vi "load_class-file.vi"(8 "error in (no error)":errorcluster, 11 "class_path":path) -> (0 "error out":errorcluster)   [LabVIEW 2015, in "lv-dialog.lvlib" / "v1.lvlib"]
uses:
  v1.lvlib
  private/_controls/fg_command.ctl
  class/v1.lvclass
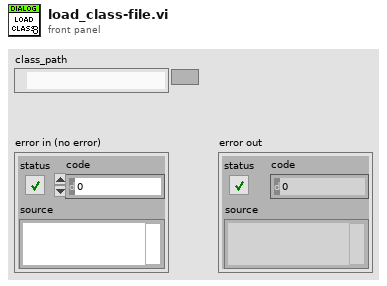
[diagram p1: front panel]
types:
  T1 = typedef "lv-dialog.lvlib/v1.lvlib/fg_command.ctl" = enum16{"null", "initialize", "read", "write", "shutdown"}
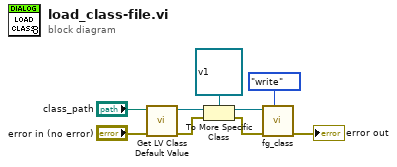
[diagram p0: block diagram]
diagram:
  n1 = call <vilib>:"Get LV Class Default Value.vi"("error in (no error)"="error in (no error)", "class path"="class_path") -> ("error out"=w2:errorcluster, "object"=w3:refnum<class>)  [unwired: 8 in]
  n2 = To More Specific Class(target class=refnum<class "v1.lvclass"> refnum ("lv-dialog.lvlib:v1.lvclass"), reference=w3, error in=w2) -> (specific class reference=w8:refnum<class "v1.lvclass">, error out=w7:errorcluster)
  n3 = call "fg_class.vi"("fg_command"=fg_command."write", "error in (no error)"=w7, "class in"=w8) -> ("error out"=→"error out":errorcluster)  [unwired: 7 in, 1 out]
